vi "daq_stop.vi"(8 "error in":errorcluster, 11 "Tasks":T1) -> (0 "error out":errorcluster)   [LabVIEW 2010]
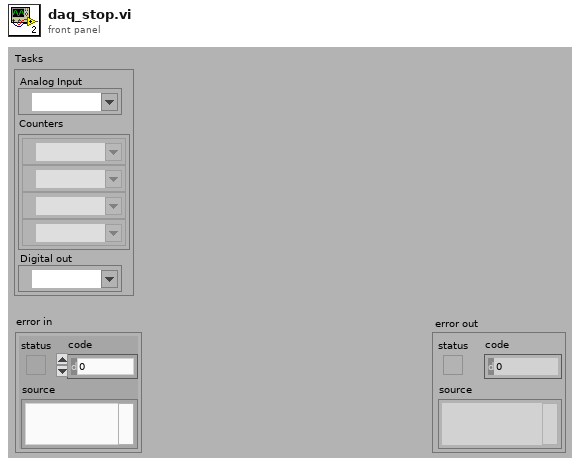
[diagram p1: front panel]
types:
  T1 = cluster{"Analog Input":refnum<k21>, "Counters":refnum<k21>[], "Digital out":refnum<k21>}
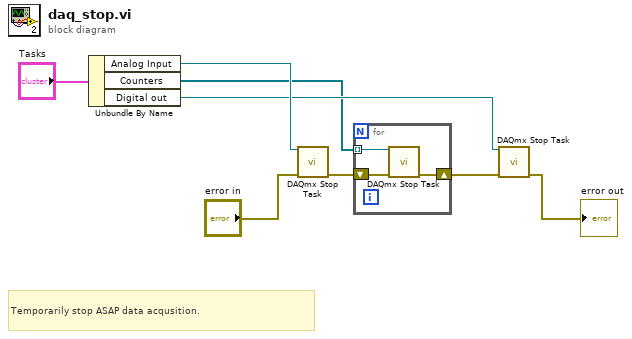
[diagram p0: block diagram]
diagram:
  # "Temporarily stop ASAP data acqusition."
  n1 = Unbundle By Name("Tasks") -> ("Analog Input"=w7:refnum<k21>, "Counters"=w1:refnum<k21>[], "Digital out"=w3:refnum<k21>)
  n2 = call <vilib>:"DAQmx Stop Task.vi"("task/channels in"=w7, "error in"="error in") -> ("error out"=w5:errorcluster)  [unwired: 13 out]
  n3 = for {
    shift-right: [w10] -> w2
    shift-left: w5 -> [w11]
    tunnel: w1 -> [w9] mode=indexing
    n4 = call <vilib>:"DAQmx Stop Task.vi"("task/channels in"=w9, "error in"=w11) -> ("error out"=w10:errorcluster)  [unwired: 13 out]
  }
  n5 = call <vilib>:"DAQmx Stop Task.vi"("task/channels in"=w3, "error in"=w2) -> ("error out"=→"error out":errorcluster)  [unwired: 13 out]
